vi "Stop Core.vi"(10 "final error code":i32, 11 "Tracer-V in":refnum<class "Tracer-V.lvclass">) -> (3 "Tracer-V out":refnum<class "Tracer-V.lvclass">)   [LabVIEW 2013, in "Tracer-V.lvclass"]
doc: "(<B>Filename</B>: Actor Framework.lvlib:Actor.lvclass:Stop Core.vi)\n\nDefines what the actor does before it stops. Use the <B>final error code</B> input to determine whether the actor shut down in response to an error.\n\nBy default, this method does nothing. A descendant class may override it to define behavior, such as shutting down any processes the actor initiated in its override of the Actor Core method."
uses:
  Tracer-V.lvclass
  Tracer-V.lvclass/Tracer-V.ctl
  Logical Systems/Tracer/Tracer.lvclass
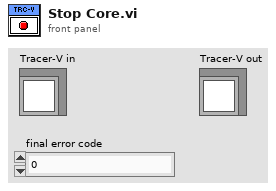
[diagram p1: front panel]
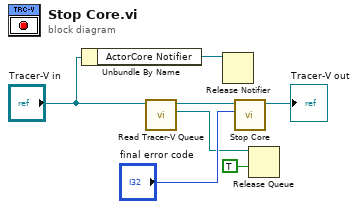
[diagram p0: block diagram]
diagram:
  n1 = Unbundle By Name("Tracer-V in") -> ("ActorCore Notifier"=w1:refnum<notifier>)
  n2 = call-dynamic "Read Tracer-V Queue.vi"("Tracer-V in"="Tracer-V in") -> ("TraceMessage Queue"=w4:refnum<queue>, "Tracer-V out"=w5:refnum<class "Tracer-V.lvclass">)  [unwired: 8 in, 1 out]
  n3 = Release Notifier(notifier=w1) -> ()  [unwired: 2 in, 3 out]
  n4 = call-parent "Stop Core.vi"("final error code"="final error code", "Actor in"=w5) -> ("Actor out"=→"Tracer-V out":refnum<class "Tracer-V.lvclass">)  [unwired: 9 in]
  n5 = Release Queue(queue=w4, force destroy? (F)=TRUE) -> ()  [unwired: 1 in, 3 out]
